vi "THzTime_SPEED_control_TA_170202.vi"(1 "ESP300 Axis":i8=1, 2 "ESP300 Address":string="1", 4 "Lockin Address":string="12") -> ()   [LabVIEW 2010]
panel:
  in  "Delay btw Pos":u32=10000
  in  "?":bool
  in  "# of Avg":i32=20
  in  "Sample Pos":dbl=-35.7
  in  "Reference Pos":dbl=6.0
  in  "SHOT202 Axis":u8=1
  in  "SHOT202 Address":string="8"
  out "Y position":dbl=-0.2690666666666667 format="%#.3p"
  out "X position":dbl=-0.49996666666666667 format="%#.3p"
  out "Power meter":dbl=48.71333333333333 format="%#.3p"
  in  "Save File Name":string="ref_sam_"
  in  "Launch server?":bool
  in  "Authorize?":bool=TRUE
  in  "CONEX-PSD9 Instrument Key 2":string="CONEX-PSD (A6ULD73M)"
  in  "Interdelay (ms)":dbl=20.0
  in  "pre delay(ms)":dbl=300.0
  out "Lock-in Y-Channel":dbl=3.63801e-12 format="%#.3p"
  out "Lock-in X-Channel":dbl=-3.4561e-11 format="%#.3p"
  out "THz Time-domain Signal Wave":cluster{"x-axis":sgl[], "y-axis":dbl[]}(graph)={"x-axis"=[-14.5, -14.51, -14.52, -14.53, -14.54, -14.55, -14.56, -14.57, -14.58, -14.59, -14.6, -14.61], "y-axis"=[1.819e-12, 1.819e-12, 0.0, 0.0, -1.819e-12, -7.27601e-12, -9.095e-12, -1.0914e-11, -1.6371e-11, -2.0009e-11, -2.1828e-11, -2.91041e-11]}
  in  "Autosave Directory for Long-term Average Scan":path=path "D:/taianh/Measurement Data/170202 Ref Sam"
  out "Phase":cluster{"f0":dbl, "df":dbl, "magnitude":dbl[]}(graph)={"f0"=0.0, "df"=1.2500000776102165, "magnitude"=[3.141592653589793, -1.3089969389957472, -1.0471975511965976, -0.7853743215168053, -0.5235987755982988, -0.2617993877991496]}
  in  "OK Button":bool
  out "Data Type":string="outp ? 1"
  in  "Enum":enum16{"X", "Y", "Abs"}(ring)
  in  "Draw":bool
  in  "Exit Program":bool
  out "Amplitude":cluster{"f0":dbl, "df":dbl, "magnitude":dbl[]}(graph)={"f0"=0.0, "df"=1.2500000776102165, "magnitude"=[14.555000066757202, 0.027320482020821914, 0.01414212213673943, 0.009999990466099009, 0.008164958022559074, 0.007320501094308238]}
  in  "Short term \nAverage#":i8=1
  in  "Step":sgl=0.005 min=0 max=10000 format="%.3f"
  in  "End Position":sgl=-18.0 min=-75 max=75 format="%#.3f"
  in  "Start Position":sgl=-14.5 min=-75 max=75 format="%#.3f"
  # "THz Experiment"
  # "Data"
  # "Auto-offset"
  # "Start Position (mm)"
  # "End Position (mm)"
  # "Step (mm)"
  # "Point Avg"
  # "# of Avg"
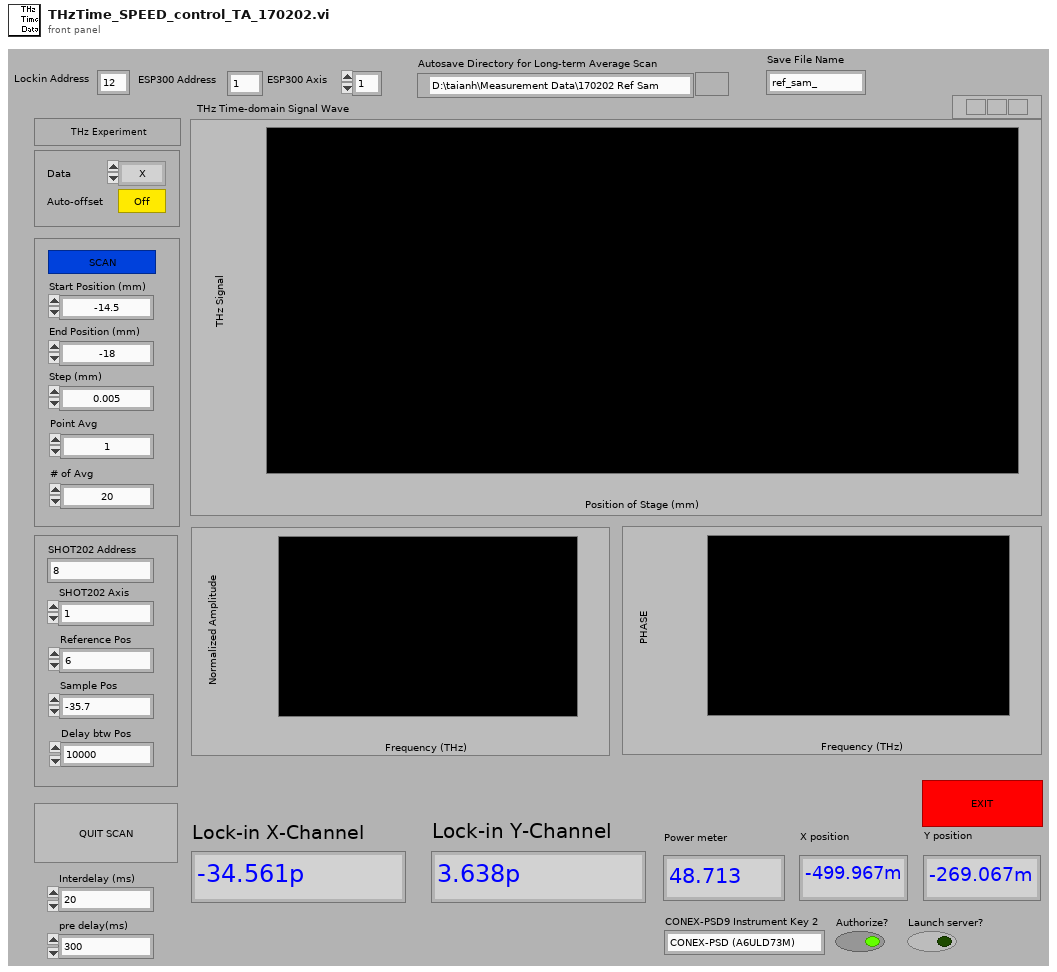
[diagram p1: front panel]
types:
  T1 = cluster{"ConexPSD Reference":refnum<k24>, "error out":errorcluster, "Component ID":i32}
  T2 = cluster{"Step Number":i32, "Step":sgl, "Start Position":sgl, "Time-out":i32, "Lockin Address":string, "Short term \nAverage#":i8, i32, "ESP300 Axis":i8, "Value":string, "pre delay(ms)":dbl, "Interdelay (ms)":dbl, "Autosave Directory for Long-term Average Scan":path, cluster{"ConexPSD Reference":refnum<k24>, "error out":errorcluster, "Component ID":i32}}
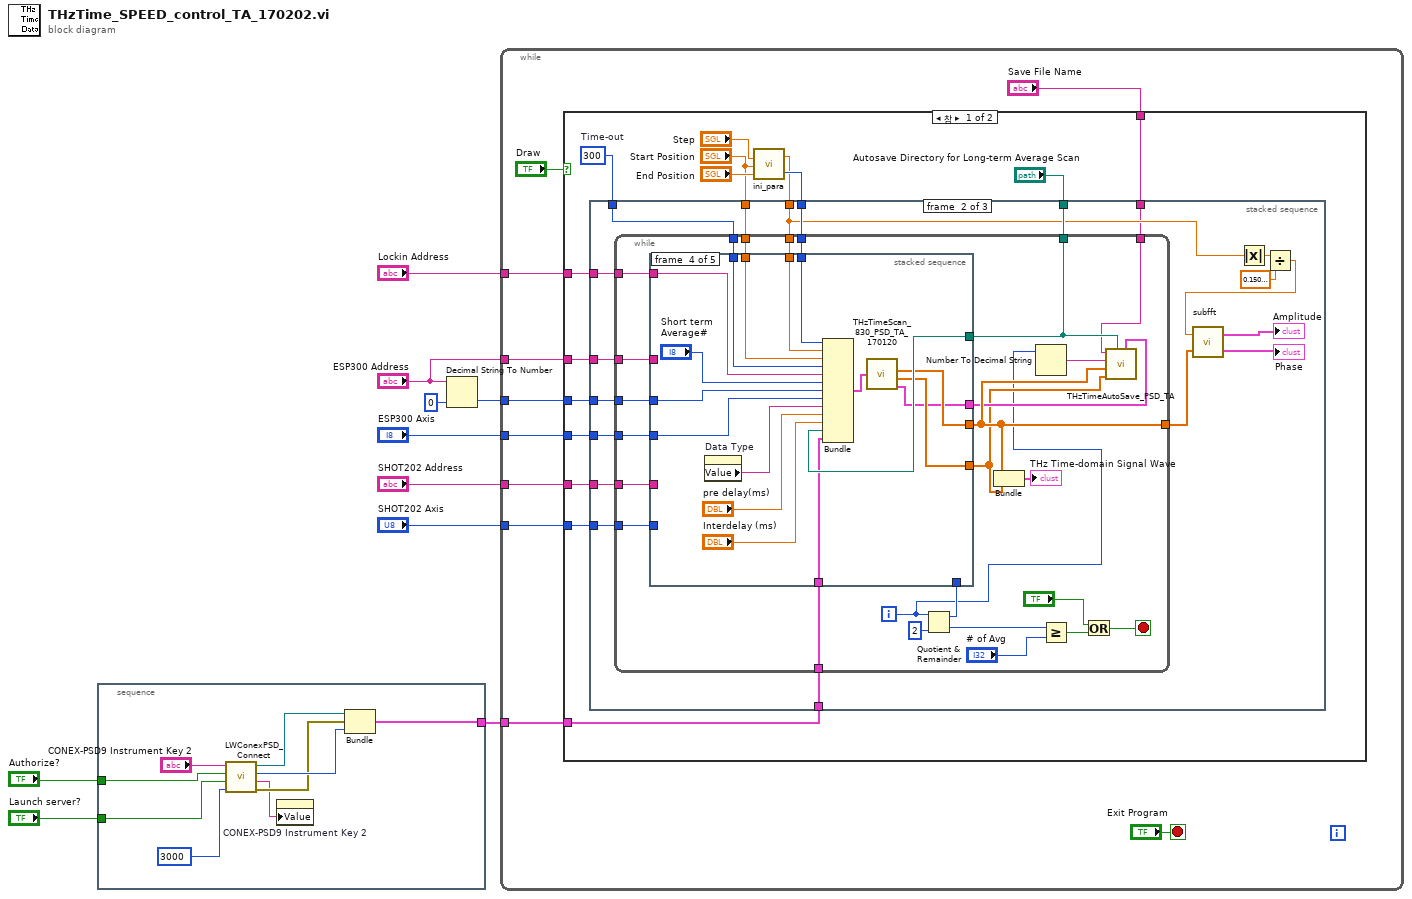
[diagram p0: block diagram]
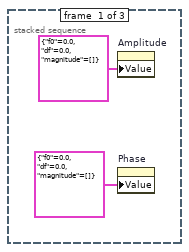
[diagram p2: hidden frame]
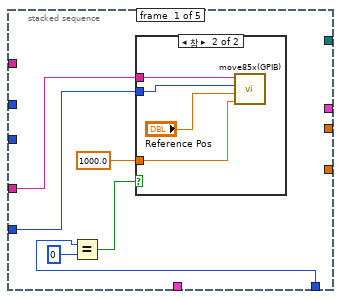
[diagram p3: hidden frame]
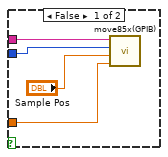
[diagram p4: hidden frame]
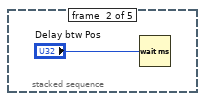
[diagram p5: hidden frame]
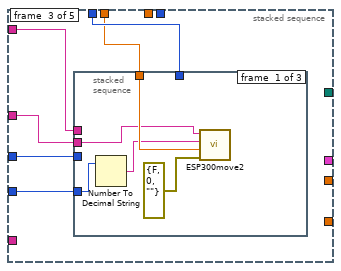
[diagram p6: hidden frame]
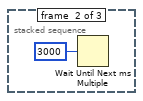
[diagram p7: hidden frame]
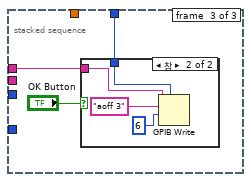
[diagram p8: hidden frame]
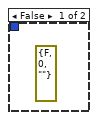
[diagram p9: hidden frame]
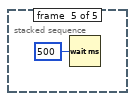
[diagram p10: hidden frame]
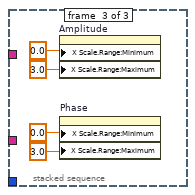
[diagram p11: hidden frame]
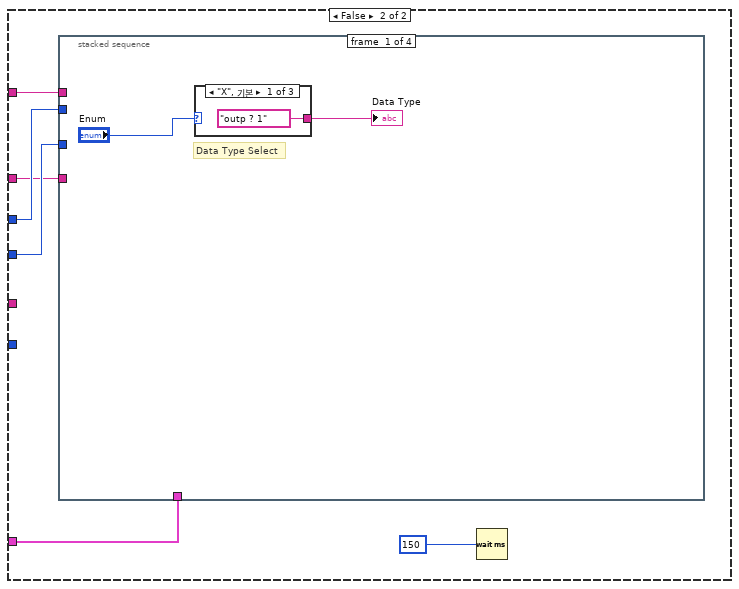
[diagram p12: hidden frame]
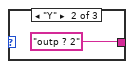
[diagram p13: hidden frame]
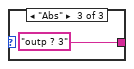
[diagram p14: hidden frame]
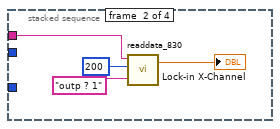
[diagram p15: hidden frame]
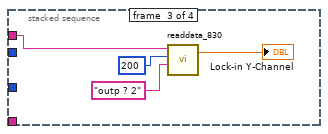
[diagram p16: hidden frame]
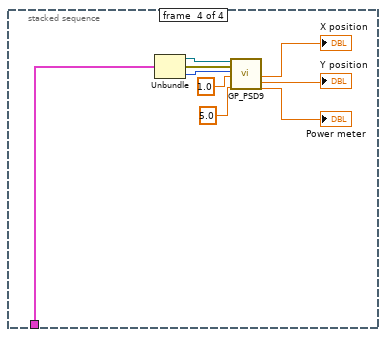
[diagram p17: hidden frame]
diagram:
  n1 = stacked-sequence {
    tunnel: "Authorize?" -> [w13]
    tunnel: [w12] -> w3
    tunnel: "Launch server?" -> [w11]
    frame #0 {
      n2 = call "LWConexPSD_Connect.vi"("DiscoverTimeout (10000 msec)"=3000, "Launch server? (True)"=w11, "Authorize? (True)"=w13, "Instrument Key"="CONEX-PSD9 Instrument Key 2") -> ("error out"=w17:errorcluster, "Instrument Key out"=w15:string, "Component ID"=w18:i32, "ConexPSD Reference"=w16:refnum<k24>)
      n3 = property on="CONEX-PSD9 Instrument Key 2" class="Str"("Value"=w15) -> ()  [unwired: 2 in, 2 out]
      n4 = Bundle("ConexPSD Reference"=w16, "error out"=w17, "Component ID"=w18) -> (w12:T1)  [unwired: 1 in]
    }
  }
  n5 = Decimal String To Number(string="ESP300 Address", default (0L)=0 ("default (0 I32)")) -> (number=w8:i32)  [unwired: 1 in, 1 out]
  n6 = while {
    tunnel: "ESP300 Axis" -> [w27]
    tunnel: "Lockin Address" -> [w26]
    tunnel: w8 -> [w25]
    tunnel: "ESP300 Address" -> [w24]
    tunnel: w3 -> [w23]
    tunnel: "SHOT202 Address" -> [w21]
    tunnel: "SHOT202 Axis" -> [w20]
    stop <- "Exit Program" stop-if-true
    n7 = case shown="참" "Draw" {
      tunnel: w26 -> [w44 w151]
      tunnel: w27 -> [w43 w153]
      tunnel: w25 -> [w42 w152]
      tunnel: w24 -> [w34 w149]
      tunnel: w23 -> [w33 w148]
      tunnel: "Save File Name" -> [w32 _]
      tunnel: w21 -> [w31 _]
      tunnel: w20 -> [w30 _]
      frame True {
        w41 = 300  # Time-out
        n8 = call "ini_para.vi"("End Position"="End Position", "Start Position"="Start Position", "Step"="Step") -> ("Step Number"=w38:i32, "Step"=w37:sgl)
        n9 = stacked-sequence {
          tunnel: w44 -> [_ w65 _]
          tunnel: w41 -> [_ w64 _]
          tunnel: w43 -> [_ w63 _]
          tunnel: w42 -> [_ w62 _]
          tunnel: w38 -> [_ w60 _]
          tunnel: w37 -> [_ w54 _]
          tunnel: "Start Position" -> [_ w61 _]
          tunnel: "Autosave Directory for Long-term Average Scan" -> [_ w59 _]
          tunnel: w34 -> [_ w52 _]
          tunnel: w33 -> [_ w51 _]
          tunnel: w32 -> [_ w50 _]
          tunnel: w31 -> [_ w48 _]
          tunnel: w30 -> [_ w47 _]
          frame #0 {
            n10 = property on="Amplitude" class="WFGraph (엄격한)"("Value"=cluster{"f0":dbl, "df":dbl, "magnitude":dbl[]} {"f0"=0.0, "df"=0.0, "magnitude"=[]} ("Spectrum")) -> ()  [unwired: 2 in, 2 out]
            n11 = property on="Phase" class="WFGraph (엄격한)"("Value"=cluster{"f0":dbl, "df":dbl, "magnitude":dbl[]} {"f0"=0.0, "df"=0.0, "magnitude"=[]} ("Spectrum")) -> ()  [unwired: 2 in, 2 out]
          }
          frame #1 {
            n12 = while {
              tunnel: w64 -> [w90]
              tunnel: w65 -> [w91]
              tunnel: w63 -> [w89]
              tunnel: w62 -> [w88]
              tunnel: w61 -> [w87]
              tunnel: w54 -> [w86]
              tunnel: w60 -> [w85]
              tunnel: w59 -> [w79]
              tunnel: [w80] -> w49
              tunnel: w52 -> [w83]
              tunnel: w51 -> [w82]
              tunnel: w50 -> [w78]
              tunnel: w48 -> [w73]
              tunnel: w47 -> [w72]
              i -> [w66]
              stop <- w69 stop-if-true
              n13 = Quotient & Remainder(x=w66, y=2) -> (x-y*floor(x/y)=w74:i32, floor(x/y)=w71:i32)
              n14 = stacked-sequence {
                tunnel: w91 -> [_ _ w112 w138 _]
                tunnel: w90 -> [_ _ w111 w139 _]
                tunnel: w89 -> [_ _ w110 w135 _]
                tunnel: w88 -> [_ _ w109 w136 _]
                tunnel: w87 -> [_ _ w108 w140 _]
                tunnel: w86 -> [_ _ _ w141 _]
                tunnel: w85 -> [_ _ _ w142 _]
                tunnel: [_ _ _ w129 _] -> w80
                tunnel: [_ _ _ w128 _] -> w76
                tunnel: w83 -> [_ _ w107 _ _]
                tunnel: w79 -> [_ _ _ w131 _]
                tunnel: w82 -> [_ _ _ w130 _]
                tunnel: [_ _ _ w127 _] -> w77
                tunnel: w74 -> [w97 _ _ _ _]
                tunnel: w73 -> [w94 _ _ _ _]
                tunnel: w72 -> [w93 _ _ _ _]
                frame #0 {
                  n15 = Equal?(x=w97, y=0) -> (x = y?=w95:bool)
                  n16 = case shown="참" w95 {
                    tunnel: w94 -> [w101 w105]
                    tunnel: w93 -> [w100 w104]
                    tunnel: 1000.0 ("wait time(ms)") -> [w98 w103]
                    frame False {
                      n17 = call "move85x(GPIB).vi"("wait time(ms)"=w98, "Moving Distance (mm) : resolutino is 1um"="Sample Pos", "Axis Number"=w100, "SHOT202 Address"=w101) -> ()
                    }
                    frame True {
                      n18 = call "move85x(GPIB).vi"("wait time(ms)"=w103, "Moving Distance (mm) : resolutino is 1um"="Reference Pos", "Axis Number"=w104, "SHOT202 Address"=w105) -> ()
                    }
                  }
                }
                frame #1 {
                  n19 = Wait (ms)(milliseconds to wait="Delay btw Pos") -> ()  [unwired: 1 out]
                }
                frame #2 {
                  n20 = stacked-sequence {
                    tunnel: w112 -> [_ _ w120]
                    tunnel: w111 -> [_ _ w119]
                    tunnel: w110 -> [w114 _ _]
                    tunnel: w109 -> [_ _ _]
                    tunnel: w108 -> [w117 _ _]
                    tunnel: w107 -> [w115 _ _]
                    frame #0 {
                      n21 = Number To Decimal String(number=w114) -> (decimal integer string=w113:string)  [unwired: 1 in]
                      n22 = call "ESP300move2.vi"("ESP300 Address"=w115, "ESP300 Channel"=w113, "Target"=w117, "error in (no error) 2"=errorcluster {"status"=FALSE, "code"=0, "source"=""}) -> ()  [unwired: 6 in, 1 out]
                    }
                    frame #1 {
                      n23 = Wait Until Next ms Multiple(millisecond multiple=3000) -> ()  [unwired: 1 out]
                    }
                    frame #2 {
                      n24 = case shown="참" "OK Button" {
                        tunnel: w120 -> [_ w125]
                        tunnel: w119 -> [_ w123]
                        frame False {
                          (unwired) errorcluster {"status"=FALSE, "code"=0, "source"=""} ("error in")
                        }
                        frame True {
                          n25 = GPIB Write(0:w125, 1:"aoff 3" ("data"), 2:i16 6 ("mode (0)"), 4:w123) -> ()  [unwired: 1 in, 2 out]
                        }
                      }
                    }
                  }
                }
                frame #3 {
                  n26 = property on="Data Type" class="Str"() -> ("Value"=w134:string)  [unwired: 2 in, 2 out]
                  n27 = Bundle("Step Number"=w142, "Step"=w141, "Start Position"=w140, "Time-out"=w139, "Lockin Address"=w138, "Short term \nAverage#"="Short term \nAverage#", w136, "ESP300 Axis"=w135, "Value"=w134, "pre delay(ms)"="pre delay(ms)", "Interdelay (ms)"="Interdelay (ms)", "Autosave Directory for Long-term Average Scan"=w131, w130) -> (w126:T2)  [unwired: 1 in]
                  n28 = call "THzTimeScan_830_PSD_TA_170120.vi"("input"=w126) -> ("x-axis"=w129:sgl[], "y-axis"=w128:dbl[], "ext. out"=w127:cluster{dbl[], dbl[], dbl[], dbl[], string[]})  [unwired: 1 out]
                }
                frame #4 {
                  n29 = Wait (ms)(milliseconds to wait=u32 500) -> ()  [unwired: 1 out]
                }
              }
              n30 = Bundle("x-axis"=w80, "y-axis"=w76) -> (→"THz Time-domain Signal Wave":cluster{"x-axis":sgl[], "y-axis":dbl[]})  [unwired: 1 in]
              n31 = Number To Decimal String(number=w66) -> (decimal integer string=w81:string)  [unwired: 1 in]
              n32 = Greater Or Equal?(x=w71, y="# of Avg") -> (x >= y?=w68:bool)
              n33 = Or(x="?", y=w68) -> (x .or. y?=w69:bool)
              n34 = call "THzTimeAutoSave_PSD_TA.vi"("ext. out"=w77, "Autosave Directory for Long-term Average Scan"=w79, "y-axis"=w76, "x-axis"=w80, "String"=w81, "SaveFile name"=w78) -> ()  [unwired: 4 in]
            }
            n35 = Absolute Value(x=w54) -> (abs(x)=w55:sgl)
            n36 = Divide(x=w55, y=sgl 0.15) -> (x/y=w53:sgl)
            n37 = call "subfft.vi"("y-signal"=w49, "time step"=w53) -> ("Phase"=→"Phase":cluster{"f0":dbl, "df":dbl, "real part":dbl[]}, "Amplitude"=→"Amplitude":cluster{"f0":dbl, "df":dbl, "real part":dbl[]})
          }
          frame #2 {
            n38 = property on="Amplitude" class="WFGraph (엄격한)"("X Scale.Range:Minimum"=0.0 ("X Scale.Range:Maximum"), "X Scale.Range:Maximum"=3.0) -> ()  [unwired: 2 in, 2 out]
            n39 = property on="Phase" class="WFGraph (엄격한)"("X Scale.Range:Minimum"=0.0, "X Scale.Range:Maximum"=3.0) -> ()  [unwired: 2 in, 2 out]
          }
        }
      }
      frame False {
        n40 = stacked-sequence {
          tunnel: w153 -> [_ _ _ _]
          tunnel: w152 -> [_ _ _ _]
          tunnel: w151 -> [_ w162 w166 _]
          tunnel: w149 -> [_ _ _ _]
          tunnel: w148 -> [_ _ _ w167]
          frame #0 {
            # "Data Type Select"
            n41 = case shown="\"X\", 기본" "Enum" {
              tunnel: ["outp ? 1" "outp ? 2" "outp ? 3"] -> w155
              frame "X", Default {
              }
              frame "Y" {
              }
              frame "Abs" {
              }
            }
            "Data Type" <- w155
          }
          frame #1 {
            n42 = call "readdata_830.vi"("Command"="outp ? 1", "timeout"=200, "Lockin Address"=w162) -> ("Data"=→"Lock-in X-Channel":dbl)  [unwired: 1 in, 1 out]
          }
          frame #2 {
            n43 = call "readdata_830.vi"("Command"="outp ? 2", "timeout"=200, "Lockin Address"=w166) -> ("Data"=→"Lock-in Y-Channel":dbl)  [unwired: 1 in, 1 out]
          }
          frame #3 {
            n44 = Unbundle(w167) -> ("ConexPSD Reference"=w175:refnum<k24>, "error out"=w174:errorcluster, "Component ID"=w173:i32)
            n45 = call "GP_PSD9.vi"("ConexPSD Reference"=w175, "error out"=w174, "Component ID"=w173, "Adress"=1.0 ("shot average"), "shot average"=5.0) -> ("PositionX"=→"X position":dbl, "PositionY"=→"Y position":dbl, "LaserPower"=→"Power meter":dbl)  [unwired: 8 in, 4 out]
          }
        }
        n46 = Wait (ms)(milliseconds to wait=u32 150) -> ()  [unwired: 1 out]
      }
    }
  }
